vi "Do.vi"(8 "error in (no error)":errorcluster, 10 "Actor in":refnum<class "Actor.lvclass">, 11 "Logging Stopped Msg":refnum<class "Logging Stopped Msg.lvclass">) -> (0 "error out":errorcluster, 2 "Actor out":refnum<class "Actor.lvclass">)   [LabVIEW 2024, in "Automation Controller.lvlib" / "Logging Stopped Msg.lvclass"]
doc: "This VI delivers the message to the actor by calling the appropriate method(s) on the actor."
uses:
  Logging Stopped Msg.lvclass
  <vilib>/ActorFramework/Actor/Actor.lvclass
  89ddd6a9-8b6b-4689-b228-f69b822ce328.vi
  Automation Controller/Automation Controller.lvclass
  Logging Stopped Msg.lvclass/Logging Stopped Msg.ctl
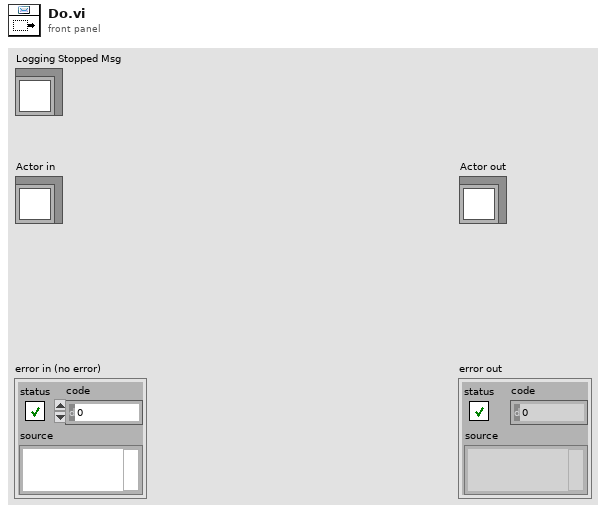
[diagram p1: front panel]
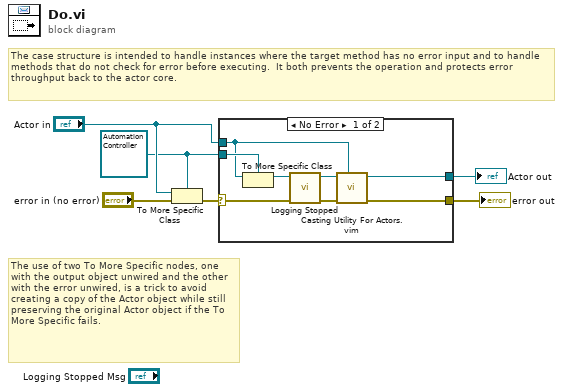
[diagram p0: block diagram]
diagram:
  w2 = refnum<class "Automation Controller.lvclass"> refnum ("Actor in")
  # "The use of two To More Specific nodes, one with the output object unwired and the other with the error unwired, is a trick to avoid creating a copy of the Actor object while still preserving the original Actor object if the To More Specific fails."
  # "The case structure is intended to handle instances where the target method has no error input and to handle methods that do not check for error before executing.  It both prevents the operation and protects error throughput back to the actor core."
  n1 = To More Specific Class(target class=w2, reference="Actor in", error in="error in (no error)") -> (error out=w1:errorcluster)  [unwired: 1 out]
  n2 = case shown="No Error" w1 {
    selector: w1 -> [w14 w16]
    tunnel: [w9 w16] -> w6
    tunnel: [w10 w15] -> w5
    tunnel: "Actor in" -> [w11 w15]
    tunnel: w2 -> [w12 _]
    frame No Error {
      n3 = To More Specific Class(target class=w12, reference=w11) -> (specific class reference=w13:refnum<class "Automation Controller.lvclass">)  [unwired: 1 in, 1 out]
      n4 = call-dynamic "Logging Stopped.vi"("error in (no error)"=w14, "Automation Controller in"=w13) -> ("error out"=w8:errorcluster, "State Machine Acto out"=w7:refnum<class "State Machine Actor.lvclass">)  [unwired: 8 in]
      n5 = call "Casting Utility For Actors.vim"("type"=w11, "error in (no error)"=w8, "Actor in"=w7) -> ("error out"=w9:errorcluster, "Actor out"=w10:refnum<class "Actor.lvclass">)  [unwired: 7 in]
    }
    frame Error {
      # "If type check fails, pass the original object out again."
    }
  }
  "error out" <- w6
  "Actor out" <- w5
